vi "Resize.vi"(8 "error in (no error)":errorcluster, 11 "MainController in":refnum<class "MainController.lvclass">) -> (0 "error out":errorcluster, 3 "MainController out":refnum<class "MainController.lvclass">)   [LabVIEW 2012, in "Win8uiFramework.lvlib" / "MainController.lvclass"]
uses:
  MainController.lvclass
  ViewableActor.lvclass/ViewableActor.ctl
  MainController.lvclass/MainController.ctl
  Read Main Pane.vi
  Read Active SubPanel.vi
  Read Inactive SubPanel.vi
  Read UI VI Ref.vi
  Read AppBar SubPanel.vi
  Read Charm SubPanel.vi
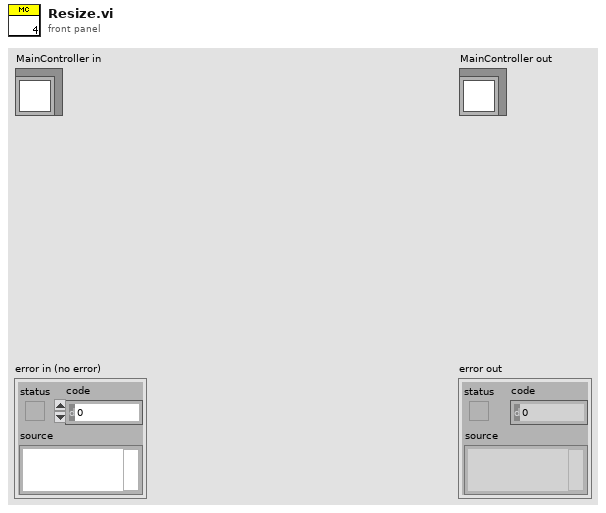
[diagram p1: front panel]
types:
  T1 = typedef "LVBoundsTypeDef.ctl" = cluster{"Width":u32, "Height":u32}
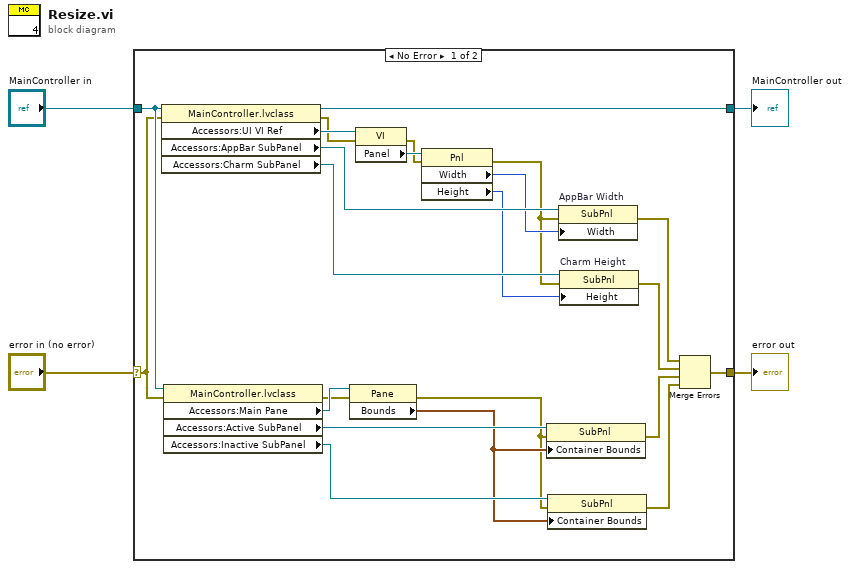
[diagram p0: block diagram]
diagram:
  n1 = case shown="No Error" "error in (no error)" {
    selector: "error in (no error)" -> [w8 w29]
    tunnel: [w18 w29] -> w3
    tunnel: [w27 w28] -> w1
    tunnel: "MainController in" -> [w17 w28]
    frame No Error {
      n2 = property class="MainController.lvclass"(reference=w17, error in=w8) -> (reference out=w27:refnum<class "MainController.lvclass">, error out=w22:errorcluster, "Accessors:UI VI Ref"=w24:refnum<vi>, "Accessors:AppBar SubPanel"=w25:refnum<vi>, "Accessors:Charm SubPanel"=w26:refnum<vi>)
      n3 = property class="MainController.lvclass"(reference=w17, error in=w8) -> (error out=w7:errorcluster, "Accessors:Main Pane"=w9:refnum<vi>, "Accessors:Active SubPanel"=w16:refnum<vi>, "Accessors:Inactive SubPanel"=w15:refnum<vi>)  [unwired: 1 out]
      n4 = property class="Pane"(reference=w9, error in=w7) -> (error out=w5:errorcluster, "Bounds"=w6:T1)  [unwired: 1 out]
      n5 = property class="VI"(reference=w24, error in=w22) -> (error out=w21:errorcluster, "Panel"=w23:refnum<vi>)  [unwired: 1 out]
      n6 = property class="Pnl"(reference=w23, error in=w21) -> (error out=w12:errorcluster, "Width"=w13:u32, "Height"=w14:u32)  [unwired: 1 out]
      n7 = property class="SubPnl"(reference=w16, error in=w5, "Container Bounds"=w6) -> (error out=w11:errorcluster)  [unwired: 1 out]
      n8 = property class="SubPnl"(reference=w15, error in=w5, "Container Bounds"=w6) -> (error out=w10:errorcluster)  [unwired: 1 out]
      n9 = property on="AppBar Width" class="SubPnl"(reference=w25, error in=w12, "Width"=w13) -> (error out=w19:errorcluster)  [unwired: 1 out]
      n10 = property on="Charm Height" class="SubPnl"(reference=w26, error in=w12, "Height"=w14) -> (error out=w20:errorcluster)  [unwired: 1 out]
      n11 = Merge Errors(w19, w20, w11, w10) -> (w18:errorcluster)
    }
    frame Error {
    }
  }
  "error out" <- w3
  "MainController out" <- w1
